vi "Calibration Accuracy.vi"(8 "error in (no error)":errorcluster, 9 "Frequency (20)":dbl=20.0 min=20.0 max=1000000.0 format="%.2f", 10 "Zone (0)":i16 min=0 max=9, 11 "VISA resource name":refnum<visa-resource-name>) -> (0 "error out":errorcluster, 1 "Radcal":dbl format="%.3f", 2 "Acal":dbl format="%.3f", 3 "VISA resource name out":refnum<visa-resource-name>)   [LabVIEW 2015, in "Agilent 428X Series.lvlib"]
doc: "This VI computes the calibration accuracy Acal and Theta Cal.\n\nDisclaimer: All accuracy calculation VI's are not part of the original \n driver. They are provided for supplementry purpose only.\n If user desires very high accuracy data, please do or \n check the calculation seperately."
uses:
  Agilent 428X Series.lvlib
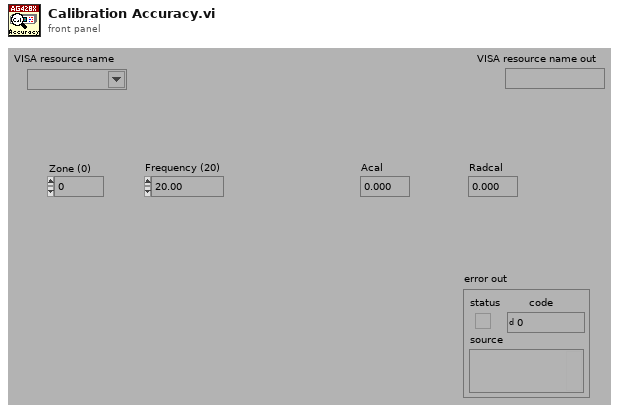
[diagram p1: front panel]
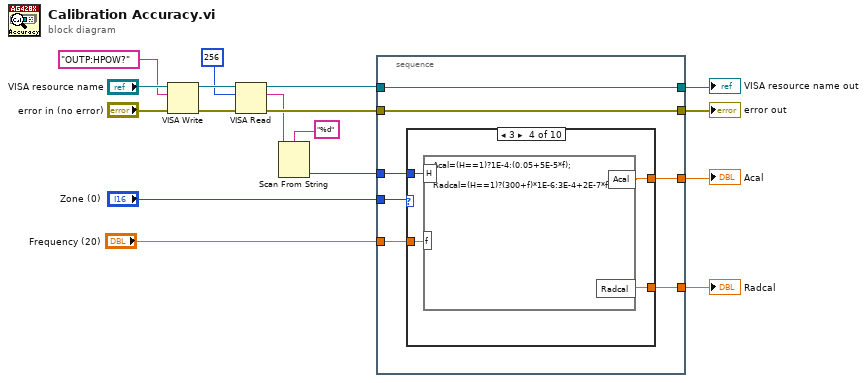
[diagram p0: block diagram]
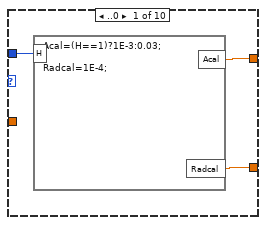
[diagram p2: hidden frame]
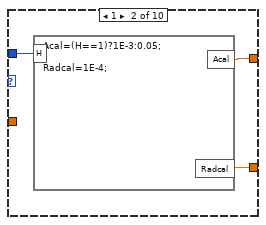
[diagram p3: hidden frame]
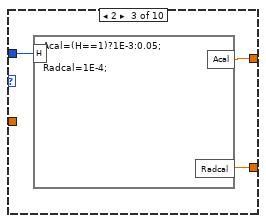
[diagram p4: hidden frame]
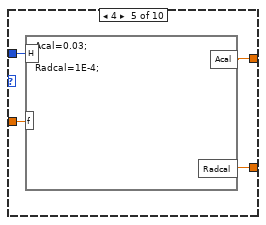
[diagram p5: hidden frame]
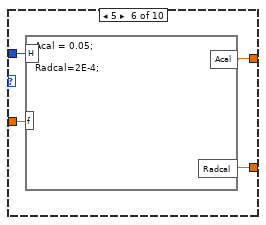
[diagram p6: hidden frame]
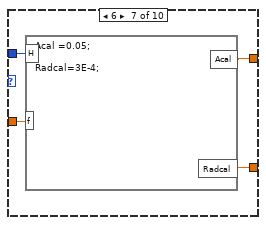
[diagram p7: hidden frame]
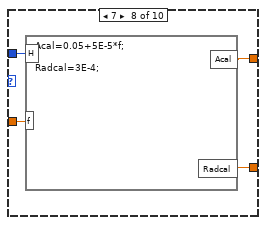
[diagram p8: hidden frame]
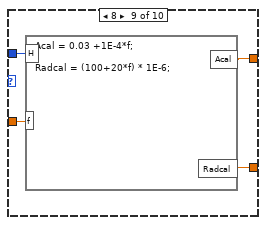
[diagram p9: hidden frame]
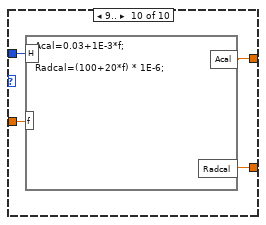
[diagram p10: hidden frame]
diagram:
  n1 = VISA Write(VISA resource name="VISA resource name", write buffer="OUTP:HPOW?" ("write buffer (\"\")"), error in (no error)="error in (no error)") -> (VISA resource name out=w12:refnum<visa-resource-name>, error out=w11:errorcluster)  [unwired: 1 out]
  n2 = VISA Read(VISA resource name=w12, byte count=u32 256 ("byte count (0)"), error in (no error)=w11) -> (VISA resource name out=w9:refnum<visa-resource-name>, read buffer=w6:string, error out=w8:errorcluster)  [unwired: 1 out]
  n3 = Scan From String(format string="%d", input string=w6) -> (output 1=w4:i32)  [unwired: 3 in, 3 out]
  n4 = stacked-sequence {
    tunnel: w9 -> [w24]
    tunnel: [w24] -> w17
    tunnel: w8 -> [w23]
    tunnel: [w23] -> w16
    tunnel: "Zone (0)" -> [w22]
    tunnel: w4 -> [w21]
    tunnel: [w20] -> w3
    tunnel: [w19] -> w2
    tunnel: "Frequency (20)" -> [w18]
    frame #0 {
      n5 = case shown="3" w22 {
        tunnel: w21 -> [w27 w30 w33 w37 w41 w45 w49 w53 w57 w61]
        tunnel: [w26 w29 w32 w36 w40 w44 w48 w52 w56 w60] -> w20
        tunnel: [w25 w28 w31 w35 w39 w43 w47 w51 w55 w59] -> w19
        tunnel: w18 -> [_ _ _ w34 w38 w42 w46 w50 w54 w58]
        frame ..0 {
          n6 = formula code="Acal=(H==1)?1E-3:0.03;\n\nRadcal=1E-4;"("H"=w27) -> ("Acal"=w26:dbl, "Radcal"=w25:dbl)
        }
        frame 1 {
          n7 = formula code="Acal=(H==1)?1E-3:0.05;\n\nRadcal=1E-4;"("H"=w30) -> ("Acal"=w29:dbl, "Radcal"=w28:dbl)
        }
        frame 2 {
          n8 = formula code="Acal=(H==1)?1E-3:0.05;\n\nRadcal=1E-4;"("H"=w33) -> ("Acal"=w32:dbl, "Radcal"=w31:dbl)
        }
        frame 3 {
          n9 = formula code="Acal=(H==1)?1E-4:(0.05+5E-5*f);\n\nRadcal=(H==1)?(300+f)*1E-6:3E-4+2E-7*f;"("H"=w37, "f"=w34) -> ("Acal"=w36:dbl, "Radcal"=w35:dbl)
        }
        frame 4 {
          n10 = formula code="Acal=0.03;\n\nRadcal=1E-4;"("H"=w41, "f"=w38) -> ("Acal"=w40:dbl, "Radcal"=w39:dbl)
        }
        frame 5 {
          n11 = formula code="Acal = 0.05;\n\nRadcal=2E-4;"("H"=w45, "f"=w42) -> ("Acal"=w44:dbl, "Radcal"=w43:dbl)
        }
        frame 6 {
          n12 = formula code="Acal =0.05;\n\nRadcal=3E-4;"("H"=w49, "f"=w46) -> ("Acal"=w48:dbl, "Radcal"=w47:dbl)
        }
        frame 7 {
          n13 = formula code="Acal=0.05+5E-5*f;\n\nRadcal=3E-4;"("H"=w53, "f"=w50) -> ("Acal"=w52:dbl, "Radcal"=w51:dbl)
        }
        frame 8 {
          n14 = formula code="Acal = 0.03 +1E-4*f;\n\nRadcal = (100+20*f) * 1E-6;"("H"=w57, "f"=w54) -> ("Acal"=w56:dbl, "Radcal"=w55:dbl)
        }
        frame 9.. {
          n15 = formula code="Acal=0.03+1E-3*f;\n\nRadcal=(100+20*f) * 1E-6;"("H"=w61, "f"=w58) -> ("Acal"=w60:dbl, "Radcal"=w59:dbl)
        }
      }
    }
  }
  "VISA resource name out" <- w17
  "error out" <- w16
  "Acal" <- w3
  "Radcal" <- w2
